vi "Create Element.vi"(9 "Attributes":refnum<class "Attribute.lvclass">[](array[class]), 10 "uid":string, 11 "class":string) -> (3 "Element":refnum<class "Element.lvclass">)   [LabVIEW 2023, in "VILab.lvlib" / "Element.lvclass"]
uses:
  Element.lvclass
  Attribute.lvclass
  Element.lvclass/Element.ctl
  Reference/Reference.lvclass
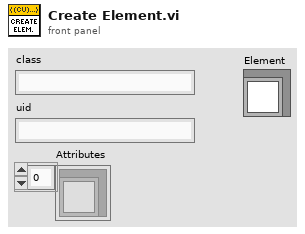
[diagram p1: front panel]
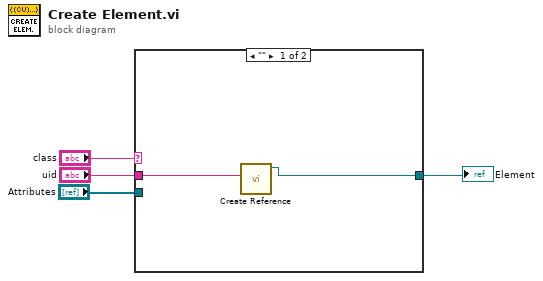
[diagram p0: block diagram]
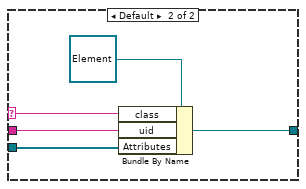
[diagram p2: hidden frame]
diagram:
  n1 = case shown="\"\"" "class" {
    selector: "class" -> [_ w10]
    tunnel: "uid" -> [w6 w9]
    tunnel: "Attributes" -> [_ w8]
    tunnel: [w5 w7] -> w1
    frame "" {
      n2 = call "Create Reference.vi"("uid"=w6) -> ("Reference"=w5:refnum<class "Reference.lvclass">)  [unwired: 10 in]
    }
    frame Default {
      n3 = Bundle By Name(cluster=refnum<class "Element.lvclass"> refnum ("VILab.lvlib:Element.lvclass"), "class"=w10, "uid"=w9, "Attributes"=w8) -> (w7:refnum<class "Element.lvclass">)
    }
  }
  "Element" <- w1
